vi "抽奖程序.vi"() -> ()   [LabVIEW 2018]
panel:
  out "数组":string[](array[string])
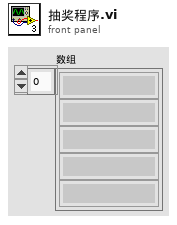
[diagram p1: front panel]
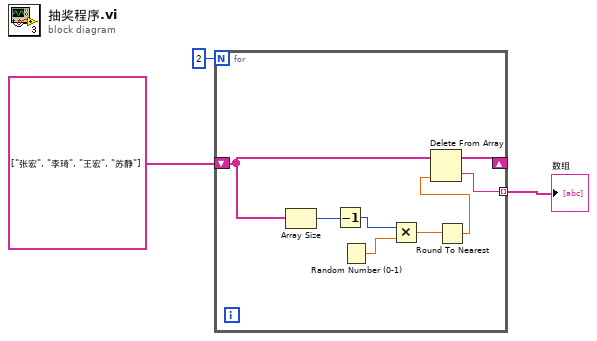
[diagram p0: block diagram]
diagram:
  n1 = for {
    N: 2 -> [_]
    shift-right: [w7] -> _
    shift-left: string[] ["张宏", "李琦", "王宏", "苏静"] -> [w11]
    tunnel: [w6] -> w1 mode=indexing
    n2 = Array Size(array=w11) -> (size(s)=w5:i32)
    n3 = Decrement(x=w5) -> (x-1=w4:i32)
    n4 = Random Number (0-1)() -> (number: 0 to 1=w10:dbl)
    n5 = Multiply(x=w4, y=w10) -> (x*y=w9:dbl)
    n6 = Round To Nearest(number=w9) -> (nearest integer value=w8:dbl)
    n7 = Delete From Array(array=w11, index=w8) -> (deleted portion=w6:string, array with subset deleted=w7:string[])  [unwired: 1 in]
  }
  "数组" <- w1
